vi "KeySight 53230A VISA Save to file.vi"() -> ()   [LabVIEW 2018]
uses:
  <instrlib>/Agilent 532XX Series/Public/Configure/Configure Channel (Basic).vi
  <instrlib>/Agilent 532XX Series/Public/Configure/Configure Channel (Voltage Range).vi
  <instrlib>/Agilent 532XX Series/Public/Configure/Configure Channel (Threshold Voltage).vi
  <instrlib>/Agilent 532XX Series/Public/Configure/Configure Channel (Slop).vi
  <instrlib>/Agilent 532XX Series/Public/Configure/Measurement/Configure Measurement (Totalize Timed).vi
  <instrlib>/Agilent 532XX Series/Public/Data/Read Measurement (Single).vi
  <instrlib>/Agilent 532XX Series/Agilent 532XX Series.lvlib
panel:
  in  "file path (use dialog)":path=path "C:/Users/User/Desktop/Counter meas/Test.txt"
  out "Number of Measurments":i32
  out "Count":dbl format="%#_12g"
  in  "stop":bool
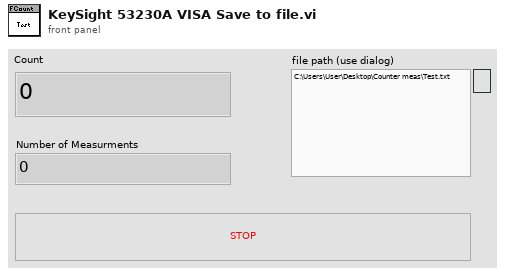
[diagram p1: front panel]
types:
  T1 = enum16{"open", "replace", "create", "open or create", "replace or create", "replace or create with confirmation"}
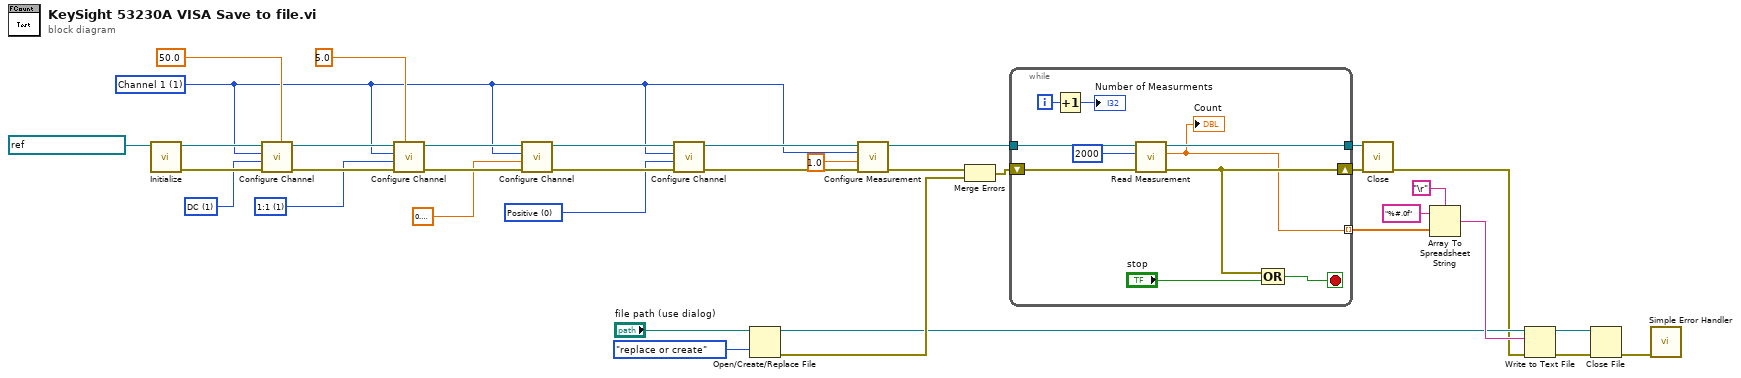
[diagram p0: block diagram]
diagram:
  w20 = 0 items=["Positive", "Negative"] ("Active Edge (1: Negative)")
  w27 = 1 items=["1:1"=1, "10:1"=10] ("Probe Factor ( 1:1)")
  w30 = 50.0 items=["50"=50.0, "1E+6"=1000000.0] ("Impedance (1E+6 Ohm)")
  w31 = 1 items=["AC", "DC"] ("Coupling (0: AC)")
  w15 = 1 items=["Channel 1"=1, "Channel 2"=2] ("Channel (1: Channel 1)")
  n1 = call <instrlib>:"Initialize.vi"("VISA resource name"=refnum<visa-resource-name> "KeySight_53230A") -> ("error out"=w34:errorcluster, "VISA resource name out"=w35:refnum<visa-resource-name>)  [unwired: 9 in]
  n2 = call-poly <instrlib>:"Configure Channel.vi"("Impedance (1E+6 Ohm)"=w30, "error in (no error)"=w34, "Coupling (0: AC)"=w31, "Channel (1: Channel 1)"=w15, "VISA resource name"=w35) -> ("error out"=w29:errorcluster, "VISA resource name out"=w28:refnum<visa-resource-name>)  [unwired: 5 in]
  n3 = call-poly <instrlib>:"Configure Channel.vi"("Voltage Range (5V)"=5.0, "error in (no error)"=w29, "Probe Factor ( 1:1)"=w27, "Channel (1: Channel 1)"=w15, "VISA resource name"=w28) -> ("error out"=w25:errorcluster, "VISA resource name out"=w23:refnum<visa-resource-name>)  [unwired: 5 in]
  n4 = call-poly <instrlib>:"Configure Channel.vi"("error in (no error)"=w25, "Threshold Voltage (0 V)"=0.30000000000000004, "Channel (1: Channel 1)"=w15, "VISA resource name"=w23) -> ("error out"=w21:errorcluster, "VISA resource name out"=w22:refnum<visa-resource-name>)  [unwired: 6 in]
  n5 = call-poly <instrlib>:"Configure Channel.vi"("error in (no error)"=w21, "Active Edge (1: Negative)"=w20, "Channel (1: Channel 1)"=w15, "VISA resource name"=w22) -> ("error out"=w17:errorcluster, "VISA resource name out"=w16:refnum<visa-resource-name>)  [unwired: 6 in]
  n6 = Open/Create/Replace File(file path (use dialog)="file path (use dialog)", operation (0:open)=T1."replace or create") -> (refnum out=w5:refnum<file>, error out=w10:errorcluster)  [unwired: 4 in, 1 out]
  n7 = call-poly <instrlib>:"Configure Measurement.vi"("error in (no error)"=w17, "Timed Totalize (0.1 s)"=1.0, "Channel (1: Channel 1)"=w15, "VISA resource name"=w16) -> ("error out"=w18:errorcluster, "VISA resource name out"=w19:refnum<visa-resource-name>)  [unwired: 6 in]
  n8 = Merge Errors(w18, w10) -> (w11:errorcluster)
  n9 = while {
    tunnel: w19 -> [w43]
    tunnel: [w42] -> w33
    shift-right: [w41] -> w32
    shift-left: w11 -> [w46]
    tunnel: [w38] -> w9 mode=indexing
    i -> [w39]
    stop <- w44 stop-if-true
    n10 = Increment(x=w39) -> (x+1=→"Number of Measurments":i32)
    n11 = call-poly <instrlib>:"Read Measurement.vi"("error in (no error)"=w46, "Timeout (10000 ms)"=u32 2000, "VISA resource name"=w43) -> ("error out"=w41:errorcluster, "Measurement"=w38:dbl, "VISA resource name out"=w42:refnum<visa-resource-name>)  [unwired: 6 in]
    "Count" <- w38
    n12 = Compound Arithmetic op=OR(w41, "stop") -> (w44:bool)
  }
  n13 = call <instrlib>:"Close.vi"("error in (no error)"=w32, "VISA resource name"=w33) -> ("error out"=w2:errorcluster)  [unwired: 9 in]
  n14 = Array To Spreadsheet String(delimiter (Tab)="\r", array=w9, 3:"%#.0f" ("format string")) -> (spreadsheet string=w6:string)
  n15 = Write to Text File(file (use dialog)=w5, text=w6, error in=w2) -> (refnum out=w3:refnum<file>, error out=w4:errorcluster)  [unwired: 1 in, 1 out]
  n16 = Close File(refnum=w3, error in=w4) -> (error out=w1:errorcluster)  [unwired: 1 out]
  n17 = call <vilib>:"Simple Error Handler.vi"("error in (no error)"=w1) -> ()  [unwired: 4 in, 5 out]
